vi "Construct.vi"(1 "Circle Shape in":refnum<class "CircleShape.lvclass">, 2 "Is Static":bool) -> (0 "Circle Collider out":refnum<class "Circle Collider.lvclass">)   [LabVIEW 2022 SP3, in "Circle Collider.lvclass"]
uses:
  Circle Collider.lvclass
  Shapes/CircleShape/CircleShape.lvclass
  Shapes/CircleShape/CircleShape.lvclass/CircleShape.ctl
  Circle Collider.lvclass/Circle Collider.ctl
  Collider/Collider.lvclass
  D:/Programowanie/Studia/Labview/CollisionSimulator/Project/Engine/Objects/Collisions/Collider/Collider.lvclass
  D:/Programowanie/Studia/Labview/CollisionSimulator/Project/Engine/Objects/Components/Component/Component.lvclass
  D:/Programowanie/Studia/Labview/CollisionSimulator/Project/Engine/Objects/Collisions/Circle Collider/Circle Collider.lvclass
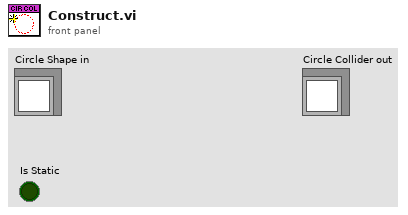
[diagram p1: front panel]
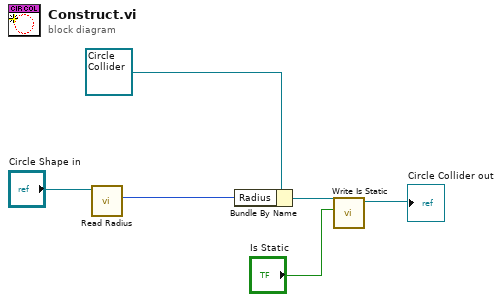
[diagram p0: block diagram]
diagram:
  n1 = call "Read Radius.vi"("CircleShape in"="Circle Shape in") -> ("Radius"=w4:i16)  [unwired: 8 in, 2 out]
  n2 = Bundle By Name(cluster=refnum<class "Circle Collider.lvclass"> refnum ("Circle Collider.lvclass"), "Radius"=w4) -> (w3:refnum<class "Circle Collider.lvclass">)
  n3 = call "Write Is Static.vi"("Is Static"="Is Static", "Collider in"=w3) -> ("Collider out"=→"Circle Collider out":refnum<class "Circle Collider.lvclass">)  [unwired: 8 in, 1 out]
